vi "SSL Data Receiver.vi"(11 "SSL Data 2":refnum<vi>) -> (2 "SSL RefBox":T1, 3 "SSL Vision":T1)   [LabVIEW 2017]
uses:
  <extravilib>/ChannelInstances/Lossy Stream-a[.](u8)/)Channel.ctl
  Control/SSL Data Control.ctl
  Control/SSL UDP Address.ctl
  Control/File Player.ctl
  <extravilib>/ChannelInstances/Lossy Stream-a[.](u8)/Write With Abort.vi
  <extravilib>/ChannelInstances/Lossy Stream-a[.](u8)/Endpoint.vi
  <extravilib>/ChannelInstances/Stream-a[.](u8)/Instantiate.vi
  <extravilib>/ChannelInstances/Lossy Stream-a[.](u8)/Instantiate.vi
  <extravilib>/ChannelInstances/Lossy Stream-a[.](u8)/)Channel.vi
  <extravilib>/ChannelInstances/Lossy Stream-a[.](u8).lvlib
panel:
  in  "Boolean 2":refnum<vi>
  in  "Cluster in":refnum<vi>
  in  "RefBox UDP RX":refnum<vi>
  in  "SSL UDP RX":refnum<vi>
  out "error out":errorcluster
  out "error out 4":errorcluster
  out "error out":errorcluster
  # "UDP"
  # "LOG"
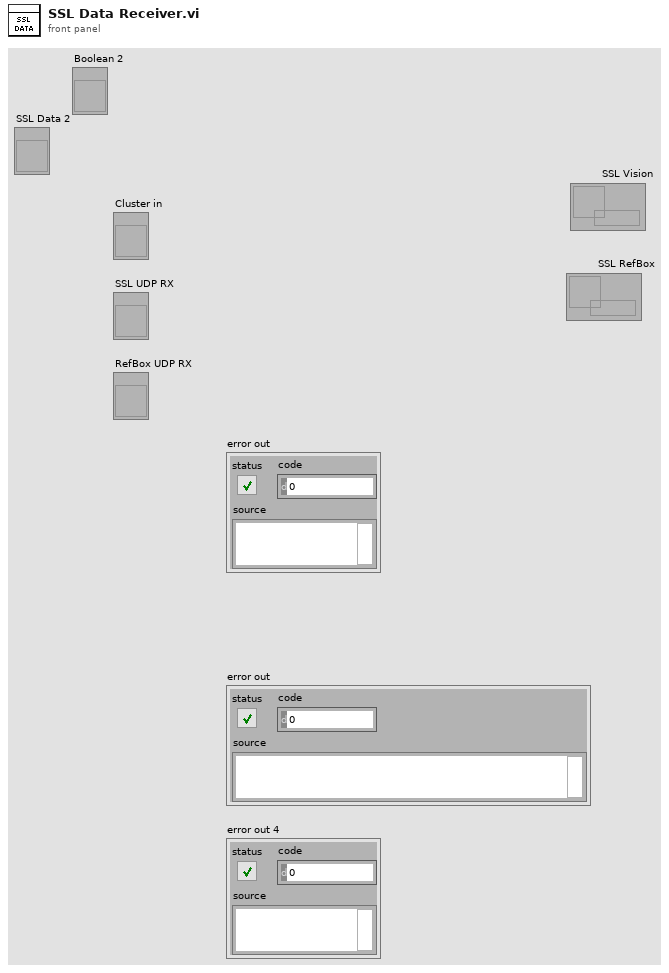
[diagram p1: front panel]
types:
  T1 = typedef "Lossy Stream-a[.](u8).lvlib/)Channel.ctl" = refnum<queue>
  T2 = typedef "Stream-a[.](u8).lvlib/)Channel.ctl" = refnum<queue>
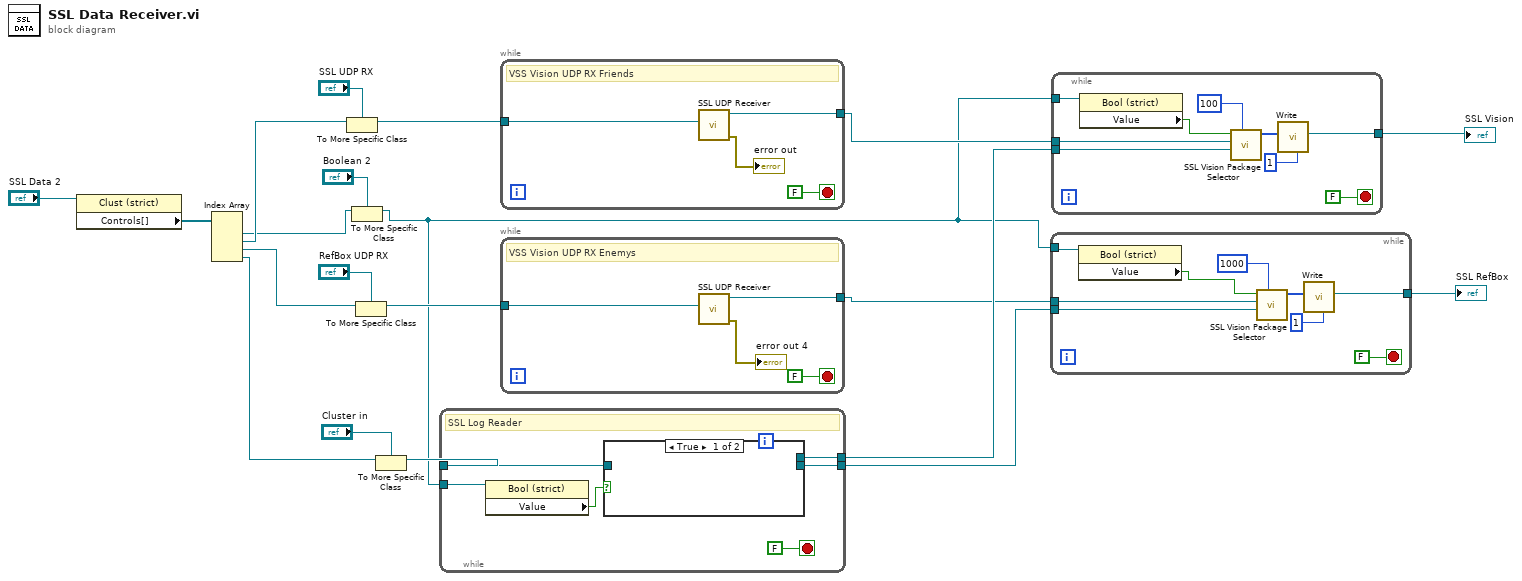
[diagram p0: block diagram]
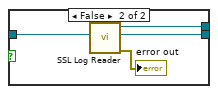
[diagram p2: hidden frame]
diagram:
  n1 = property on="Property Node" class="Clust (strict)"(reference="SSL Data 2") -> ("Controls[]"=w14:refnum<vi>[])  [unwired: 1 in, 2 out]
  n2 = Index Array(array=w14) -> (element #1=w2:refnum<vi>, element #2=w11:refnum<vi>, element #3=w8:refnum<vi>, element #4=w5:refnum<vi>)  [unwired: 4 in]
  n3 = To More Specific Class(target class="SSL UDP RX", reference=w11) -> (specific class reference=w12:refnum<vi>)  [unwired: 1 in, 1 out]
  n4 = To More Specific Class(target class="Boolean 2", reference=w2) -> (specific class reference=w1:refnum<vi>)  [unwired: 1 in, 1 out]
  n5 = To More Specific Class(target class="RefBox UDP RX", reference=w8) -> (specific class reference=w10:refnum<vi>)  [unwired: 1 in, 1 out]
  n6 = To More Specific Class(target class="Cluster in", reference=w5) -> (specific class reference=w7:refnum<vi>)  [unwired: 1 in, 1 out]
  n7 = while {
    tunnel: [w24] -> w17
    tunnel: [w25] -> w19
    tunnel: w7 -> [w23]
    tunnel: w1 -> [w22]
    stop <- FALSE stop-if-true
    # "SSL Log Reader"
    n8 = property class="Bool (strict)"(reference=w22) -> ("Value"=w21:bool)  [unwired: 1 in, 2 out]
    n9 = case shown="True" w21 {
      tunnel: [_ w29] -> w25
      tunnel: [_ w28] -> w24
      tunnel: w23 -> [_ w27]
      frame True {
      }
      frame False {
        n10 = call "SSL Log Reader.vi"("Cluster 2"=w27) -> ("error out"=→"error out":errorcluster, "channel 2"=w28:T2, "Channel out"=w29:T2)  [unwired: 7 in, 1 out]
      }
    }
  }
  n11 = while {
    tunnel: [w34] -> w20
    tunnel: w12 -> [w31]
    stop <- FALSE stop-if-true
    # "VSS Vision UDP RX Friends"
    n12 = call "SSL UDP Receiver.vi"("SSL UDP Receiver 2"=w31) -> ("error out"=→"error out":errorcluster, "Channel out"=w34:T1)  [unwired: 9 in]
  }
  n13 = while {
    tunnel: [w36] -> w18
    tunnel: w10 -> [w35]
    stop <- FALSE stop-if-true
    # "VSS Vision UDP RX Enemys"
    n14 = call "SSL UDP Receiver.vi"("SSL UDP Receiver 2"=w35) -> ("error out"=→"error out 4":errorcluster, "Channel out"=w36:T1)  [unwired: 9 in]
  }
  n15 = while {
    tunnel: w18 -> [w47]
    tunnel: w17 -> [w46]
    tunnel: [w43] -> w16
    tunnel: w1 -> [w40]
    stop <- FALSE stop-if-true
    n16 = property class="Bool (strict)"(reference=w40) -> ("Value"=w41:bool)  [unwired: 1 in, 2 out]
    n17 = call "SSL Vision Package Selector.vi"("timeout in ms (-1)"=1000, "channel in"=w46, "Channel in"=w47, "Modo"=w41) -> ("element"=w44:u8[])  [unwired: 7 in]
    n18 = call <extravilib>:"Write.vi"("size (1)"=1, "element"=w44) -> ("channel"=w43:T1)  [unwired: 7 in, 2 out]
  }
  "SSL RefBox" <- w16
  n19 = while {
    tunnel: w20 -> [w56]
    tunnel: w19 -> [w55]
    tunnel: [w52] -> w15
    tunnel: w1 -> [w50]
    stop <- FALSE stop-if-true
    n20 = property class="Bool (strict)"(reference=w50) -> ("Value"=w49:bool)  [unwired: 1 in, 2 out]
    n21 = call "SSL Vision Package Selector.vi"("timeout in ms (-1)"=100, "channel in"=w55, "Channel in"=w56, "Modo"=w49) -> ("element"=w53:u8[])  [unwired: 7 in]
    n22 = call <extravilib>:"Write.vi"("size (1)"=1, "element"=w53) -> ("channel"=w52:T1)  [unwired: 7 in, 2 out]
  }
  "SSL Vision" <- w15
